vi "Create.vi"(8 "error in (no error)":errorcluster, 10 "Handle":refnum<class "Protected Actor Handle.lvclass">) -> (0 "error out":errorcluster, 3 "Protected Actor Handle out":refnum<class "Protected Actor Handle.lvclass">)   [LabVIEW 2020, in "AF Debug.lvlib" / "Protected Actor Handle.lvclass"]
doc: "Given the information about an actor, provided by the debug layer of the Actor Framework, this VI creates an actor handle that an attached debugger can use for limited manipulation of the running actor."
uses:
  Protected Actor Handle.lvclass
  vi.lib/ActorFramework/Inspection API/Protected Actor Handle/Protected Actor Handle.lvclass
  Protected Actor Handle.lvclass/Protected Actor Handle.ctl
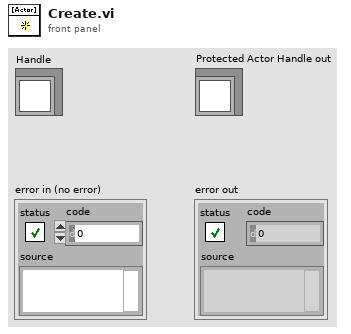
[diagram p1: front panel]
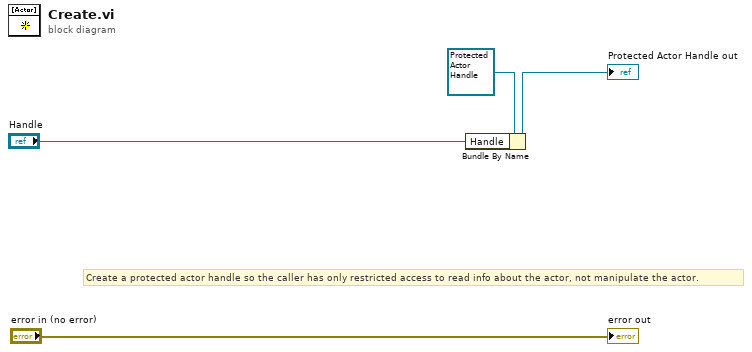
[diagram p0: block diagram]
diagram:
  # "Create a protected actor handle so the caller has only restricted access to read info about the actor, not manipulate the actor."
  n1 = Bundle By Name(cluster=refnum<class "Protected Actor Handle.lvclass"> refnum ("Protected Actor Handle in"), "Handle"="Handle") -> (→"Protected Actor Handle out":refnum<class "Protected Actor Handle.lvclass">)
  "error out" <- "error in (no error)"
